vi "Custom Trigger Windows Host.vi"() -> ()   [LabVIEW 2010]
uses:
  <vilib>/userDefined/High Color/nirio_resource_hc.ctl
  <vilib>/rvi/interface/nirviOpenFPGA/nirviOpenFPGA.xnode
  Custom Trigger AI.vi
  <vilib>/rvi/interface/nirviOpenFPGA/nirviOpenFPGA.ctl
  <vilib>/rvi/interface/nirviOpenFPGA/nirviopenstate.ctl
  <vilib>/picture/picture.llb/imagedata.ctl
  <vilib>/rvi/interface/common/nirviIntfCommonState.ctl
  <vilib>/rvi/interface/common/nirviIntfModes.ctl
  Program Files/National Instruments/LabVIEW 2010/resource/RVI/emulation/niLvFpgaEmulationMode.ctl
  <vilib>/eio/XNode/Errors/EIOXNodeErrorStruct.ctl
  <vilib>/eio/XNode/Errors/EIOXNodeInternalErrorTypes.ctl
  <vilib>/eio/XNode/Errors/EIOXNodeUserErrorTypes.ctl
  <vilib>/XNodeSupport/XNodeRect32.ctl
  <vilib>/XNodeSupport/XNodeInt.ctl
  <vilib>/XNodeSupport/XNodeTerms.ctl
  <vilib>/XNodeSupport/XNodeTerm.ctl
  <vilib>/XNodeSupport/XNodeString.ctl
  <vilib>/XNodeSupport/XNodeVariant.ctl
  <vilib>/XNodeSupport/XNodeBool.ctl
  <vilib>/rvi/interface/nirviReadWriteControl/nirviReadWriteControl.xnode
  <vilib>/rvi/interface/nirviMethod/nirviMethod.xnode
  <vilib>/rvi/interface/common/niFpgaNodeNameForErrorReporting.ctl
  <vilib>/rvi/interface/nirviCloseFPGA/nirviCloseFPGA.xnode
  <vilib>/rvi/interface/RandomDataEmulation/nirviRandomDataOpen.vi
  <vilib>/rvi/interface/RandomDataEmulation/nirviRandomDataDMAMethods.vi
  <vilib>/rvi/interface/RandomDataEmulation/nirviRandomDataClose.vi
  <vilib>/XNodeSupport/NI_XNodeSupport.lvlib
panel:
  in  "Host Read Timeout (ms)":i32=100
  in  "Stop":bool
  in  "AI Threshold Low":i16=-16000
  in  "Trigger Enable":bool
  in  "Samples to Read":i32=100
  in  "FPGA Sample Period (us)":u32=1000
  in  "AI Threshold High":i16=16000
  out "Analog Data":i16[](graph)
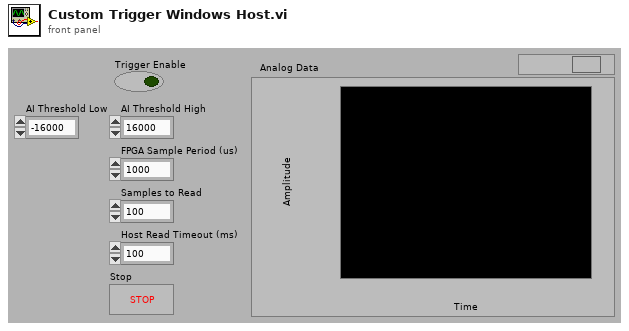
[diagram p1: front panel]
types:
  T1 = typedef "niFpgaNodeNameForErrorReporting.ctl" = enum16{"Open FPGA VI Reference", "Read/Write Control", "Invoke Method: Abort", "Invoke Method: Acknowledge IRQ", "Invoke Method: Download", "Invoke Method: FIFO.Configure", "Invoke Method: FIFO.Read", "Invoke Method: FIFO.Start", "Invoke Method: FIFO.Stop", "Invoke Method: FIFO.Write", "Invoke Method: Reset", "Invoke Method: Run", "Invoke Method: Wait on IRQ", "Close FPGA VI Reference"}
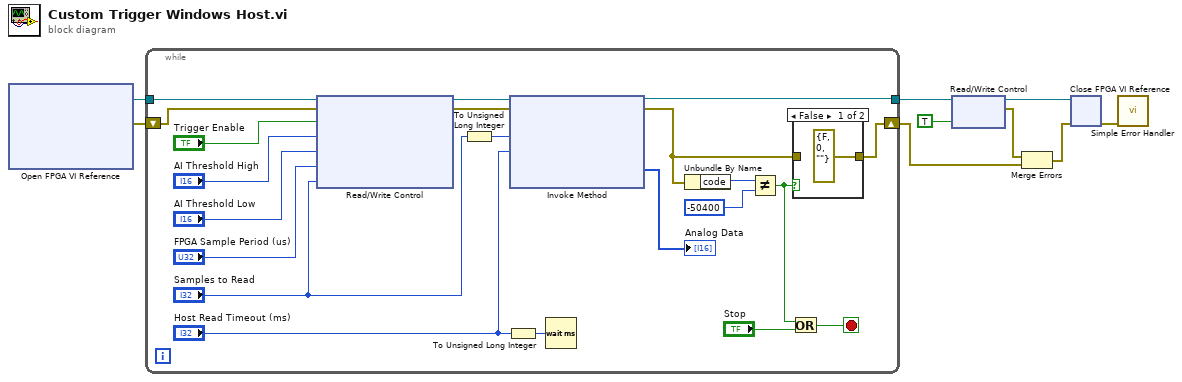
[diagram p0: block diagram]
diagram:
  n1 = xnode "Open FPGA VI Reference"() -> ("FPGA VI Reference Out"=w8:refnum<k20>, "error out"=w9:errorcluster)  [unwired: 2 in]
  n2 = while {
    tunnel: w8 -> [w26]
    tunnel: [w14] -> w6
    shift-right: [w13] -> w3
    shift-left: w9 -> [w27]
    stop <- w17 stop-if-true
    n3 = xnode "Read/Write Control"("FPGA VI Reference In"=w26, "error in"=w27, "Trigger Enable"="Trigger Enable", "AI Threshold High"="AI Threshold High", "AI Threshold Low"="AI Threshold Low", "FPGA Sample Period (us)"="FPGA Sample Period (us)", "Number of Samples"="Samples to Read") -> ("FPGA VI Reference Out"=w16:refnum<k20>, "error out"=w20:errorcluster)
    n4 = To Unsigned Long Integer(number="Samples to Read") -> (unsigned 32bit integer=w18:u32)
    n5 = To Unsigned Long Integer(number="Host Read Timeout (ms)") -> (unsigned 32bit integer=w10:u32)
    n6 = xnode "Invoke Method"("FPGA VI Reference In"=w16, "error in"=w20, "Number of Elements"=w18, "Timeout (ms)"="Host Read Timeout (ms)") -> ("FPGA VI Reference Out"=w14:refnum<k20>, "error out"=w28:errorcluster, "Data"=→"Analog Data":i16[])  [unwired: 1 out]
    n7 = Wait (ms)(milliseconds to wait=w10) -> ()  [unwired: 1 out]
    n8 = Unbundle By Name(w28) -> ("code"=w30:i32)
    n9 = Not Equal?(x=w30, y=-50400) -> (x != y?=w12:bool)
    n10 = Or(x=w12, y="Stop") -> (x .or. y?=w17:bool)
    n11 = case shown="False" w12 {
      tunnel: w28 -> [_ w61]
      tunnel: [errorcluster {"status"=FALSE, "code"=0, "source"=""} ("error out") w61] -> w13
      frame False {
      }
      frame True {
      }
    }
  }
  n12 = xnode "Read/Write Control"("FPGA VI Reference In"=w6, "Stop"=TRUE) -> ("FPGA VI Reference Out"=w5:refnum<k20>, "error out"=w2:errorcluster)  [unwired: 1 in]
  n13 = Merge Errors(w2, w3) -> (w1:errorcluster)
  n14 = xnode "Close FPGA VI Reference"("FPGA VI Reference In"=w5, "error in"=w1) -> ("error out"=w7:errorcluster)
  n15 = call <vilib>:"Simple Error Handler.vi"("error in (no error)"=w7) -> ()  [unwired: 1 in, 8 out]
